vi "CtoFandK.vi"() -> ()   [LabVIEW 2014]
panel:
  out "Fahrenheit to Kelvin":dbl
  out "Celsius to Kelvin":dbl
  out "Celsius to Fahrenheit":dbl
  out "Fahrenheit to Celsius":dbl
  in  "Celsius":dbl
  in  "Fahrenheit":dbl
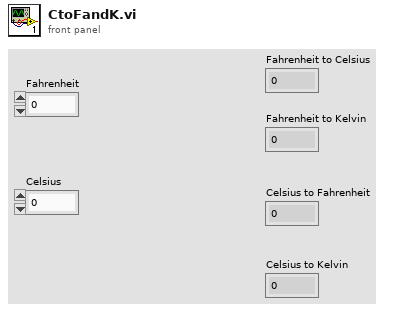
[diagram p1: front panel]
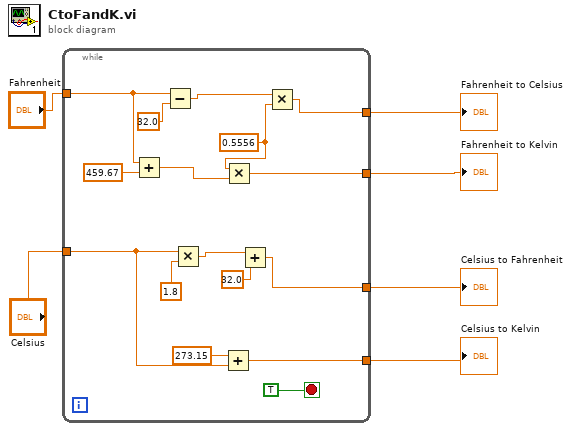
[diagram p0: block diagram]
diagram:
  n1 = while {
    tunnel: [w19] -> w6
    tunnel: [w16] -> w5
    tunnel: "Fahrenheit" -> [w14]
    tunnel: [w11] -> w3
    tunnel: "Celsius" -> [w10]
    tunnel: [w8] -> w1
    stop <- TRUE stop-if-true
    w13 = 0.5556 ("y")
    n2 = Add(x=w14, y=459.67) -> (x+y=w12:dbl)
    n3 = Subtract(x=w14, y=32.0) -> (x-y=w17:dbl)
    n4 = Multiply(x=w10, y=1.8) -> (x*y=w21:dbl)
    n5 = Add(x=273.15, y=w10) -> (x+y=w8:dbl)
    n6 = Multiply(x=w13, y=w12) -> (x*y=w11:dbl)
    n7 = Add(x=w21, y=32.0) -> (x+y=w19:dbl)
    n8 = Multiply(x=w17, y=w13) -> (x*y=w16:dbl)
  }
  "Fahrenheit to Celsius" <- w5
  "Celsius to Fahrenheit" <- w6
  "Celsius to Kelvin" <- w1
  "Fahrenheit to Kelvin" <- w3
